vi "Check-Move_user_lib.vi"(9 "message":string, 10 "Target":path, 11 "ZIP FILE":path) -> (0 "error out":errorcluster)   [LabVIEW 2014]
uses:
  <vilib>/zip/NI_Unzip.lvlib
panel:
  out "Files Transferred:":i16(slide) scale=0.0..471.0
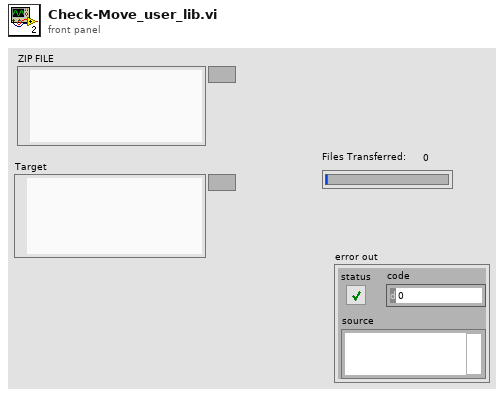
[diagram p1: front panel]
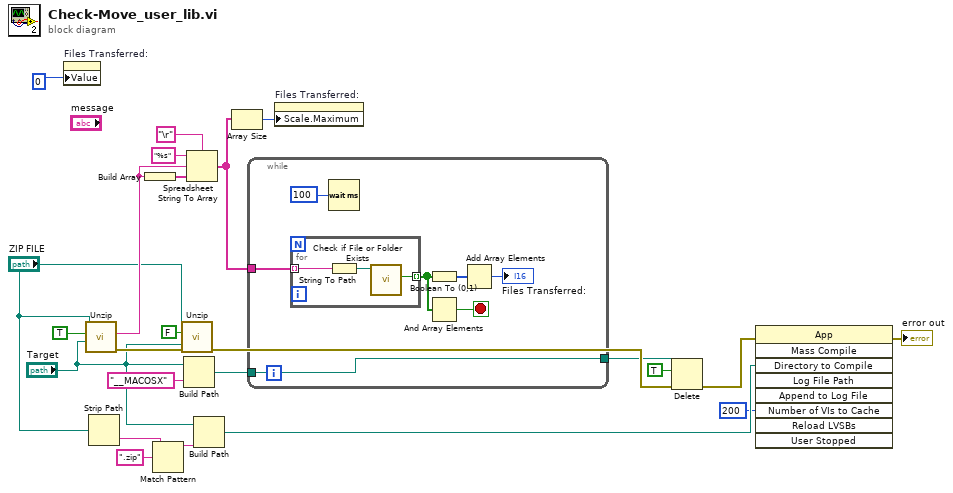
[diagram p0: block diagram]
diagram:
  n1 = property on="Files Transferred:" class="Slide (strict)"("Value"=i16 0 ("Files Transferred:")) -> ()  [unwired: 2 in, 2 out]
  n2 = call <vilib>:"Unzip.vi"("Target directory (same as Zip file if empty)"="Target", "Preview only?"=TRUE, "Zip file"="ZIP FILE") -> ("error out"=w17:errorcluster, "Preview"=w20:string)  [unwired: 6 in, 1 out]
  n3 = Strip Path(path="ZIP FILE") -> (name=w11:string)  [unwired: 1 out]
  n4 = Build Array(w20) -> (w23:string[])
  n5 = Match Pattern(string=w11, regular expression=".zip") -> (before substring=w9:string)  [unwired: 1 in, 3 out]
  n6 = call <vilib>:"Unzip.vi"("error in (no error)"=w17, "Target directory (same as Zip file if empty)"="Target", "Preview only?"=FALSE, "Zip file"="ZIP FILE") -> ("error out"=w5:errorcluster)  [unwired: 5 in, 2 out]
  n7 = Build Path(base path="Target", name or relative path="__MACOSX") -> (appended path=w3:path)
  n8 = Spreadsheet String To Array(delimiter (Tab)="\r", format string="%s", spreadsheet string=w20, array type (2D Dbl)=w23) -> (array=w18:string[])
  n9 = Build Path(base path="Target", name or relative path=w9) -> (appended path=w6:path)
  n10 = Array Size(array=w18) -> (size(s)=w19:i32)
  n11 = while {
    tunnel: w18 -> [w31]
    tunnel: [w25] -> w4
    tunnel: w3 -> [w25]
    stop <- w27 stop-if-true
    n12 = for {
      tunnel: w31 -> [w34] mode=indexing
      tunnel: [w32] -> w28 mode=indexing
      n13 = String To Path(string=w34) -> (path=w33:path)
      n14 = call <vilib>:"Check if File or Folder Exists.vi"("path"=w33) -> ("file or folder exists?"=w32:bool)  [unwired: 8 in, 2 out]
    }
    n15 = Wait (ms)(milliseconds to wait=u32 100) -> ()  [unwired: 1 out]
    n16 = Boolean To (0,1)(Boolean=w28) -> (0, 1=w29:i16[])
    n17 = And Array Elements(Boolean array=w28) -> (logical AND=w27:bool)
    n18 = Add Array Elements(numeric array=w29) -> (sum=→"Files Transferred:":i16)
  }
  n19 = property on="Files Transferred:" class="Slide (strict)"("Scale.Maximum"=w19) -> ()  [unwired: 2 in, 2 out]
  n20 = Delete(path (use dialog)=w4, entire hierarchy (F)=TRUE, error in=w5) -> (error out=w12:errorcluster)  [unwired: 2 in, 2 out]
  n21 = invoke class="App" method="Mass Compile"(error in=w12, "Directory to Compile"=w6, "Number of VIs to Cache"=u32 200) -> (error out=→"error out":errorcluster)  [unwired: 6 in, 8 out]
